vi "Save Data.vi"(8 "error in (no error)":errorcluster, 10 "signal out":waveform(dbl), 11 "Tdms in":refnum<class "Tdms.lvclass">) -> (0 "error out":errorcluster, 3 "Tdms out":refnum<class "Tdms.lvclass">)   [LabVIEW 2020, in "Tdms.lvlib" / "Tdms.lvclass"]
uses:
  Tdms.lvclass
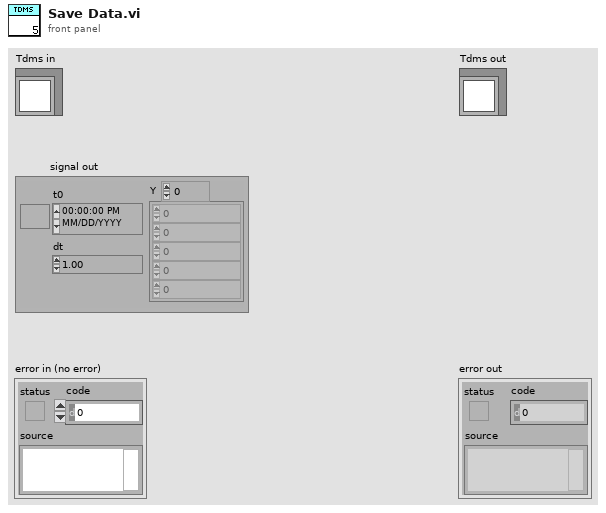
[diagram p1: front panel]
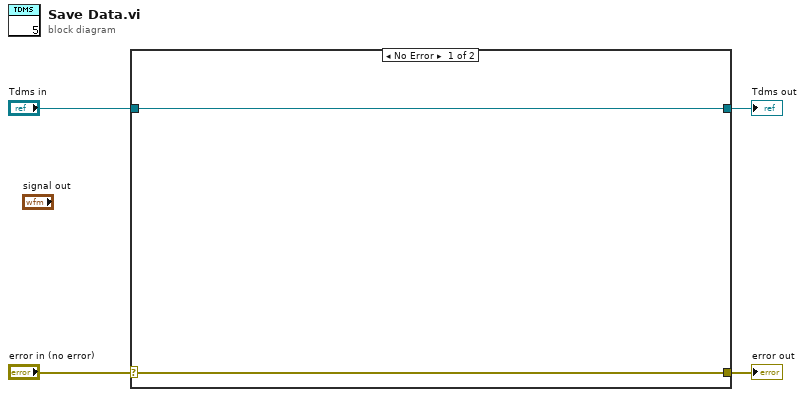
[diagram p0: block diagram]
diagram:
  n1 = case shown="No Error" "error in (no error)" {
    selector: "error in (no error)" -> [w5 w8]
    tunnel: [w5 w8] -> w3
    tunnel: [w6 w7] -> w1
    tunnel: "Tdms in" -> [w6 w7]
    frame No Error {
    }
    frame Error {
    }
  }
  "error out" <- w3
  "Tdms out" <- w1
